vi "Change Remote URL.vi"(8 "error in (no error)":errorcluster, 11 "GitPackage in":refnum<class "GitPackage.lvclass">) -> (0 "error out":errorcluster, 3 "GitPackage out":refnum<class "GitPackage.lvclass">)   [LabVIEW 2020, in "GPack.lvlib" / "GitPackage.lvclass"]
uses:
  GitPackage.lvclass
  GitPackage.lvclass/GitPackage.ctl
  <vilib>/regexp/Match Regular Expression.xnode
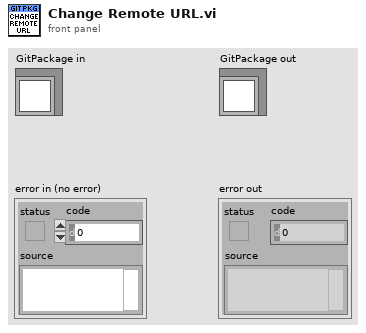
[diagram p1: front panel]
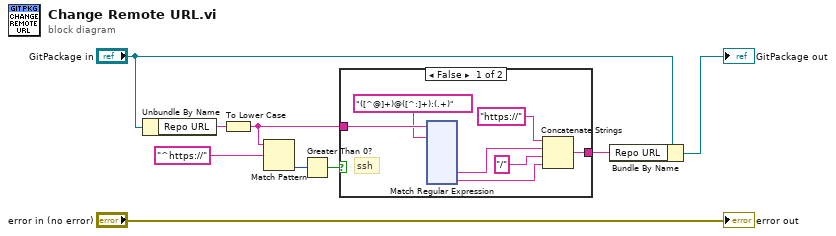
[diagram p0: block diagram]
diagram:
  n1 = Unbundle By Name("GitPackage in") -> ("Repo URL"=w8:string)
  n2 = To Lower Case(string=w8) -> (all lower case string=w4:string)
  n3 = Match Pattern(string=w4, regular expression="^https://") -> (offset past match=w6:i32)  [unwired: 1 in, 3 out]
  n4 = Greater Than 0?(x=w6) -> (x > 0?=w5:bool)
  n5 = case shown="False" w5 {
    tunnel: w4 -> [w16 w135]
    tunnel: [w10 w135] -> w3
    frame False {
      # "ssh"
      n6 = xnode "Match Regular Expression"("input string"=w16, "regular expression"="([^@]+)@([^:]+):(.+)") -> ("submatch 2"=w13:string, "submatch 3"=w11:string)  [unwired: 4 in, 6 out]
      n7 = Concatenate Strings("https://" ("string"), w13, "/" ("string"), w11) -> (w10:string)
    }
    frame True {
      # "https"
    }
  }
  n8 = Bundle By Name(cluster="GitPackage in", "Repo URL"=w3) -> (→"GitPackage out":refnum<class "GitPackage.lvclass">)
  "error out" <- "error in (no error)"
